vi "model.vi"(3 "num_iterations":i32, 4 "Y_train":dbl[][](array[numeric]), 5 "X_train":dbl[][](array[numeric])) -> ()   [LabVIEW 2020]
panel:
  out "costs":dbl[](array[numeric])
  out "Accuracy":dbl
  out "Y_predicted":dbl[][](array[numeric])
  in  "learning_rate":dbl
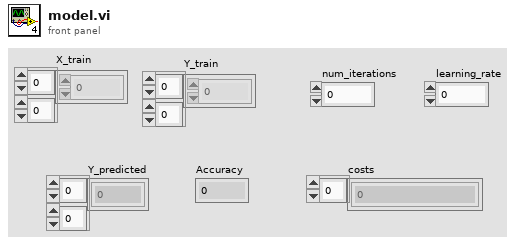
[diagram p1: front panel]
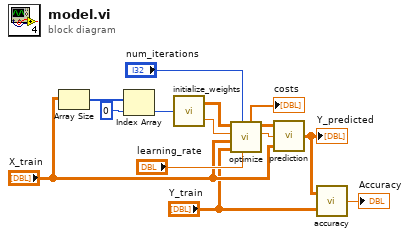
[diagram p0: block diagram]
diagram:
  n1 = Array Size(array="X_train") -> (size(s)=w14:i32[])
  n2 = Index Array(array=w14, index=0) -> (element=w12:i32)
  n3 = call "initialize_weights.vi"("dim"=w12) -> ("b"=w10:dbl, "W"=w11:dbl[][])  [unwired: 2 in]
  n4 = call "optimize.vi"("learning_rate"="learning_rate", "num_iterations"="num_iterations", "Y"="Y_train", "X"="X_train", "b"=w10, "w"=w11) -> ("trained_b"=w6:dbl, "trained_W"=w7:dbl[][], "costs"=→"costs":dbl[])  [unwired: 2 out]
  n5 = call "prediction.vi"("X"="X_train", "b"=w6, "w"=w7) -> ("Y_predicted"=w4:dbl[][])
  "Y_predicted" <- w4
  n6 = call "accuracy.vi"("Y_actual"="Y_train", "Y_predicted"=w4) -> ("Accuracy"=→"Accuracy":dbl)
